vi "load_graph.vi"() -> (1 "XY Graph":cluster{"all rows":dbl[], "all rows":dbl[]}(graph))   [LabVIEW 2025]
panel:
  out "String":string
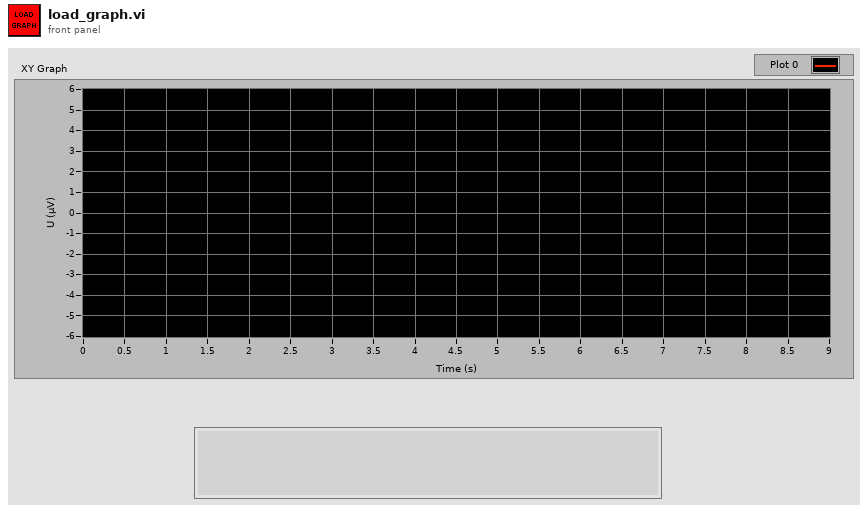
[diagram p1: front panel]
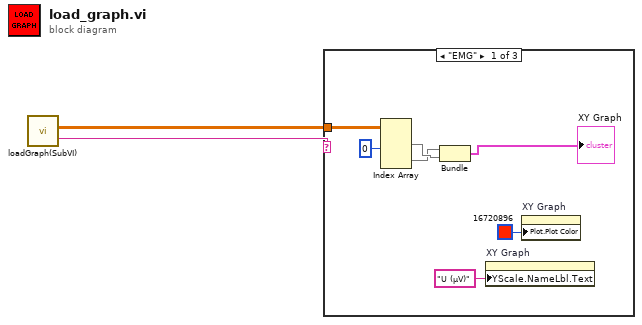
[diagram p0: block diagram]
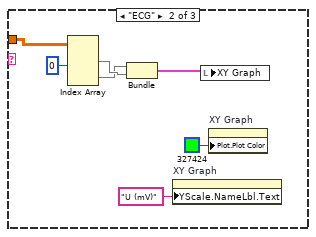
[diagram p2: hidden frame]
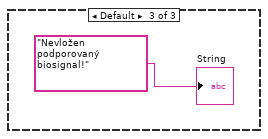
[diagram p3: hidden frame]
diagram:
  n1 = call "loadGraph(SubVI).vi"() -> ("all rows"=w2:dbl[][], "String"=w1:string)  [unwired: 10 in]
  n2 = case shown="\"EMG\"" w1 {
    tunnel: w2 -> [w7 w13 _]
    frame "EMG" {
      n3 = Index Array(array=w7, index (col) #1=0 ("disabled index (col)")) -> (element #1=w9:dbl[], element #2=w8:dbl[])  [unwired: 3 in]
      n4 = Bundle("all rows"=w8, "all rows"=w9) -> (→"XY Graph":cluster{"all rows":dbl[], "all rows":dbl[]})  [unwired: 1 in]
      n5 = property on="XY Graph" class="XYGraph (strict)"("YScale.NameLbl.Text"="U (µV)" ("Y Scale.Name Label.Text")) -> ()  [unwired: 2 in, 2 out]
      n6 = property on="XY Graph" class="XYGraph (strict)"("Plot.Plot Color"=u32 16720896) -> ()  [unwired: 2 in, 2 out]
    }
    frame "ECG" {
      n7 = Index Array(array=w13, index (col) #1=0 ("disabled index (col)")) -> (element #1=w16:dbl[], element #2=w15:dbl[])  [unwired: 3 in]
      n8 = Bundle("all rows"=w15, "all rows"=w16) -> (w12:cluster{"all rows":dbl[], "all rows":dbl[]})  [unwired: 1 in]
      n9 = property on="XY Graph" class="XYGraph (strict)"("YScale.NameLbl.Text"="U (mV)" ("Y Scale.Name Label.Text")) -> ()  [unwired: 2 in, 2 out]
      n10 = local write "XY Graph"(w12) -> ()
      n11 = property on="XY Graph" class="XYGraph (strict)"("Plot.Plot Color"=u32 327424) -> ()  [unwired: 2 in, 2 out]
    }
    frame Default {
      "String" <- "Nevložen podporovaný biosignal!"
    }
  }
